vi "Shoot SSI.vi"(10 "Robot Commands":T4={"Robot Forward-Back"=0.007874015748031496, "Robot Twist"=-0.11811023622047244, "Fire"=FALSE, "Lift/Drive Shift"=FALSE, "Raise Lifter"=FALSE, "Raise Grabber"=FALSE, "Lower Grabber"=FALSE, "Roller"=enum."DONT MOVE", "Robot Climb Both Sides"=0.0, "Grabber to Middle Position"=FALSE, "Grabber to Top Position"=FALSE, "Grabber to Bottom Position"=FALSE, "Robot Climb Left Side"=0.0, "Robot Climb Right Side"=0.0, "Speed Control Left Side"=0.0, "Speed Control Right Side"=0.0, "Lower Lifter"=FALSE, "Defense Mode"=FALSE, "Deploy Lifter"=FALSE, "Auto Targetting"=FALSE, "Do the Jiggle"=FALSE}, 11 "Shooter State":T1) -> (2 "Shoot Actuator Values Out":T2={"Catapult Winch"=0.5, "Catapult Solenoid"=enum."Reverse", "Inner LEDs"=enum."Off", "Left LEDs"=enum."Off", "Right LEDs"=enum."Off"})   [LabVIEW 2015]
uses:
  Robot Commands 2016.ctl
  Load SS/Roller State.ctl
  Shoot Actuator Values.ctl
  <vilib>/Rock Robotics/WPI/Solenoid/WPI_SolenoidValue.ctl
  Shooter Control.ctl
  Global Variables/Sensor Data.vi
  Global Variables/Temp Variables.vi
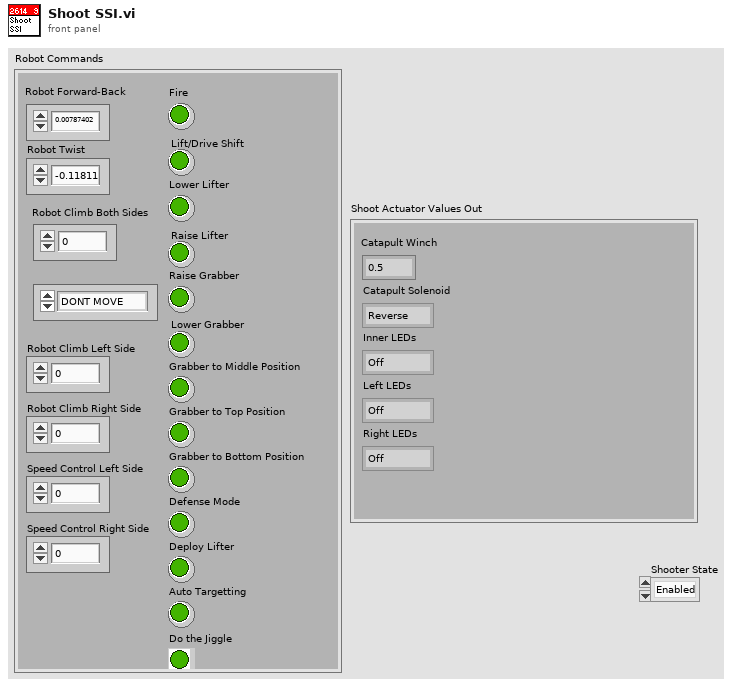
[diagram p1: front panel]
types:
  T1 = typedef "Shooter Control.ctl" = enum16{"Enabled", "Disabled"}
  T2 = typedef "Shoot Actuator Values.ctl" = cluster{"Catapult Winch":dbl, "Catapult Solenoid":T3, "Inner LEDs":T3, "Left LEDs":T3, "Right LEDs":T3}
  T3 = typedef "WPI_SolenoidValue.ctl" = enum16{"Off", "On", "Forward", "Reverse"}
  T4 = typedef "Robot Commands 2016.ctl" = cluster{"Robot Forward-Back":dbl, "Robot Twist":dbl, "Fire":bool, "Lift/Drive Shift":bool, "Raise Lifter":bool, "Raise Grabber":bool, "Lower Grabber":bool, "Roller":T5, "Robot Climb Both Sides":dbl, "Grabber to Middle Position":bool, "Grabber to Top Position":bool, "Grabber to Bottom Position":bool, "Robot Climb Left Side":dbl, "Robot Climb Right Side":dbl, "Speed Control Left Side":dbl, "Speed Control Right Side":dbl, "Lower Lifter":bool, "Defense Mode":bool, "Deploy Lifter":bool, "Auto Targetting":bool, "Do the Jiggle":bool}
  T5 = typedef "Roller State.ctl" = enum16{"DONT MOVE", "Intake", "Outtake"}
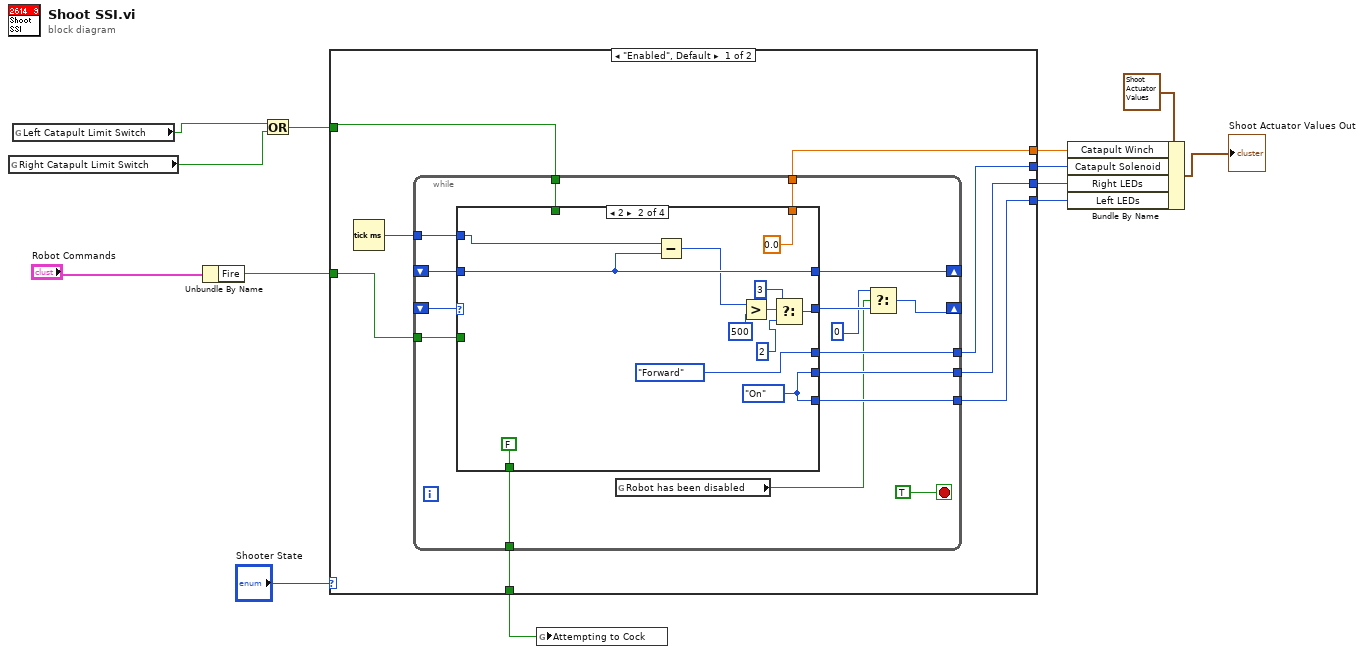
[diagram p0: block diagram]
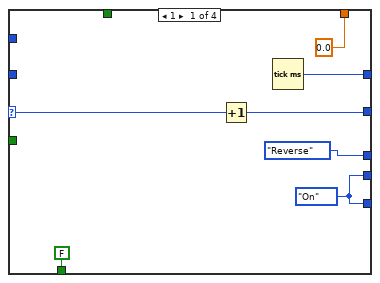
[diagram p2: hidden frame]
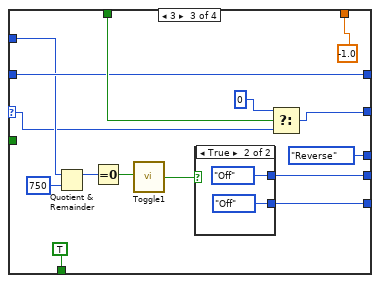
[diagram p3: hidden frame]
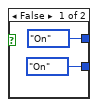
[diagram p4: hidden frame]
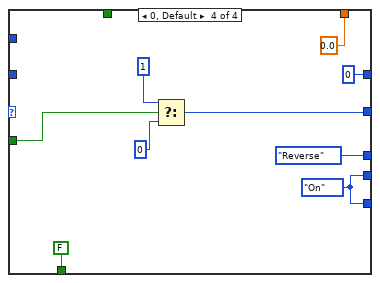
[diagram p5: hidden frame]
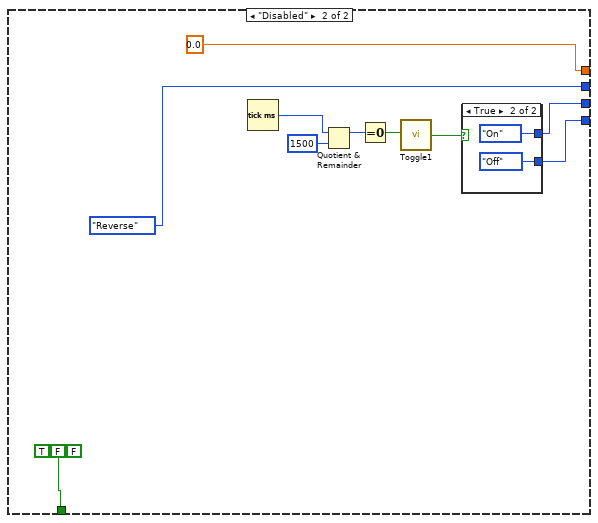
[diagram p6: hidden frame]
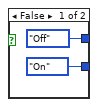
[diagram p7: hidden frame]
diagram:
  n1 = global read "Sensor Data.vi" "Right Catapult Limit Switch"() -> (w4:bool)
  n2 = global read "Sensor Data.vi" "Left Catapult Limit Switch"() -> (w5:bool)
  n3 = Unbundle By Name("Robot Commands") -> ("Fire"=w6:bool)
  n4 = Or(x=w5, y=w4) -> (x .or. y?=w7:bool)
  n5 = case shown="\"Enabled\", Default" "Shooter State" {
    tunnel: [w19 0.0] -> w10
    tunnel: w6 -> [w18 _]
    tunnel: [w20 WPI_SolenoidValue."Reverse" ("Catapult Solenoid")] -> w9
    tunnel: w7 -> [w17 _]
    tunnel: [w16 w88] -> w3
    tunnel: [w15 w87] -> w2
    tunnel: [w14 FALSE] -> w1
    frame "Enabled", Default {
      n6 = Tick Count (ms)() -> (millisecond timer value=w21:u32)
      n7 = while {
        shift-right: [w27] -> _
        shift-left: _ -> [w35]
        tunnel: [w34] -> w20
        shift-right: [w33] -> _
        shift-left: _ -> [w31]
        tunnel: w21 -> [w32]
        tunnel: [w30] -> w19
        tunnel: w18 -> [w29]
        tunnel: w17 -> [w28]
        tunnel: [w25] -> w16
        tunnel: [w24] -> w15
        tunnel: [w23] -> w14
        stop <- TRUE stop-if-true
        n8 = case shown="2" w35 {
          selector: w35 -> [w43 _ w58 _]
          tunnel: [w42 w49 w68 w82] -> w36
          tunnel: [WPI_SolenoidValue."Reverse" ("Value") WPI_SolenoidValue."Forward" ("Value") WPI_SolenoidValue."Reverse" ("Value") WPI_SolenoidValue."Reverse" ("Value")] -> w34
          tunnel: [w44 w55 w67 u32 0 ("millisecond timer value")] -> w33
          tunnel: w32 -> [_ w56 w63 _]
          tunnel: w31 -> [_ w55 w67 _]
          tunnel: [0.0 0.0 -1.0 0.0] -> w30
          tunnel: w29 -> [_ _ _ w78]
          tunnel: w28 -> [_ _ w69 _]
          tunnel: [w39 w46 w65 w77] -> w25
          tunnel: [w39 w46 w64 w77] -> w24
          tunnel: [FALSE FALSE TRUE FALSE] -> w23
          frame 1 {
            w39 = WPI_SolenoidValue."On" ("Value")
            n9 = Increment(x=w43) -> (x+1=w42:i32)
            n10 = Tick Count (ms)() -> (millisecond timer value=w44:u32)
          }
          frame 2 {
            w46 = WPI_SolenoidValue."On" ("Value")
            n11 = Subtract(x=w56, y=w55) -> (x-y=w54:u32)
            n12 = Greater?(x=w54, y=u32 500) -> (0:w52:bool)
            n13 = Select(t=3, s=w52, f=2) -> (s? t:f=w49:i32)
          }
          frame 3 {
            n14 = Quotient & Remainder(x=w63, y=u32 750) -> (x-y*floor(x/y)=w61:u32)  [unwired: 1 out]
            n15 = Equal To 0?(x=w61) -> (x = 0?=w60:bool)
            n16 = call "Toggle1.vi"("Boolean"=w60) -> ("Driver Switch 2"=w59:bool)
            n17 = case shown="True" w59 {
              tunnel: [WPI_SolenoidValue."On" ("Value") WPI_SolenoidValue."Off" ("Value")] -> w65
              tunnel: [WPI_SolenoidValue."On" ("Value") WPI_SolenoidValue."Off" ("Value")] -> w64
              frame False {
              }
              frame True {
              }
            }
            n18 = Select(t=0, s=w69, f=w58) -> (s? t:f=w68:i32)
          }
          frame 0, Default {
            w77 = WPI_SolenoidValue."On" ("Value")
            n19 = Select(t=1, s=w78, f=0) -> (s? t:f=w82:i32)
          }
        }
        n20 = global read "Temp Variables.vi" "Robot has been disabled"() -> (w22:bool)
        n21 = Select(t=0, s=w22, f=w36) -> (s? t:f=w27:i32)
      }
    }
    frame "Disabled" {
      (unwired) FALSE
      (unwired) TRUE
      n22 = Tick Count (ms)() -> (millisecond timer value=w86:u32)
      n23 = Quotient & Remainder(x=w86, y=u32 1500) -> (x-y*floor(x/y)=w91:u32)  [unwired: 1 out]
      n24 = Equal To 0?(x=w91) -> (x = 0?=w90:bool)
      n25 = call "Toggle1.vi"("Boolean"=w90) -> ("Driver Switch 2"=w89:bool)
      n26 = case shown="True" w89 {
        tunnel: [WPI_SolenoidValue."Off" ("Value") WPI_SolenoidValue."On" ("Value")] -> w88
        tunnel: [WPI_SolenoidValue."On" ("Value") WPI_SolenoidValue."Off" ("Value")] -> w87
        frame False {
        }
        frame True {
        }
      }
    }
  }
  n27 = global write "Temp Variables.vi" "Attempting to Cock"(w1) -> ()
  n28 = Bundle By Name(cluster=T2 {"Catapult Winch"=0.0, "Catapult Solenoid"=enum."Off", "Inner LEDs"=enum."Off", "Left LEDs"=enum."Off", "Right LEDs"=enum."Off"} ("Shoot Actuator Values Out 2"), "Catapult Winch"=w10, "Catapult Solenoid"=w9, "Right LEDs"=w3, "Left LEDs"=w2) -> (→"Shoot Actuator Values Out":T2)
